vi "ClientSDO_readU32.vi"(8 "error in (no error)":errorcluster, 9 "sub_index":u8, 10 "object_index":u16, 11 "ClientSDO Ref in":refnum<k24>) -> (0 "error IO":errorcluster, 1 "ErrorCode":u32, 2 "Val":u32, 3 "ClientSDO Ref out":refnum<k24>, 4 "status":i32(ring) items=["CANOPEN_OK"=0, "CANOPEN_ERROR"=-255, "CANOPEN_ERROR_ASYNC_TRANSFER_ENABLED"=-114, "CANOPEN_ASYNC_TRANSFER"=-113, "CANOPEN_ERROR_NOT_EDS_DCF_CONFIGURED"=-112, "CANOPEN_ERROR_FILE_NOT_FOUND"=-111, "CANOPEN_ERROR_NOT_IMPLEMENTED"=-110, "CANOPEN_ERROR_NO_MESSAGE"=-109, "CANOPEN_UNSUPPORTED_BITRATE"=-108, "CANOPEN_OUT_OF_CAN_INTERFACES"=-107, "CANOPEN_ERROR_DRIVER"=-106, "CANOPEN_ERROR_HW_UNDEFINED"=-105, "CANOPEN_ERROR_HW_NOT_CONNECTED"=-104, "CANOPEN_ERROR_HW_CONNECTED"=-103, "CANOPEN_ERROR_CAN_LAYER_OVRFLOW"=-102, "CANOPEN_ERROR_CAN_LAYER"=-101, "CANOPEN_CAN_LAYER_FAILED"=-100, "CANOPEN_NODE_ID_OUT_OF_RANGE"=-15, "CANOPEN_INTERNAL_STATE_ERROR"=-14, "CANOPEN_CMD_SPEC_UNKNOWN_OR_INVALLD"=-13, "CANOPEN_ERR_DEFINED_BY_APPL"=-12, "CANOPEN_OUT_OF_MEM"=-11, "CANOPEN_REMOTE_NODE_ABORT"=-10, "CANOPEN_APP_BUF_OUT_OF_RANGE"=-9, "CANOPEN_OBJECT_MISSMATCH"=-8, "CANOPEN_BUFFER_TOO_SMALL"=-7, "CANOPEN_TOGGLE"=-6, "CANOPEN_MSG_NOT_PROCESSED"=-5, "CANOPEN_TIMEOUT"=-4, "CANOPEN_UNEXPECTED_CCS"=-3, "CANOPEN_UNEXPECTED_SCS"=-2, "CANOPEN_ARG_ERROR"=-1])   [LabVIEW 2015, in "CANOpen.lvlib"]
doc: "read DWORD from <b>client </b> using SDO protocol"
uses:
  CANOpen.lvlib
  \\Mac\Home/Desktop/imt_test_app 28-06-2012/canopenlib_cli.dll
  canopenlib_cli.dll
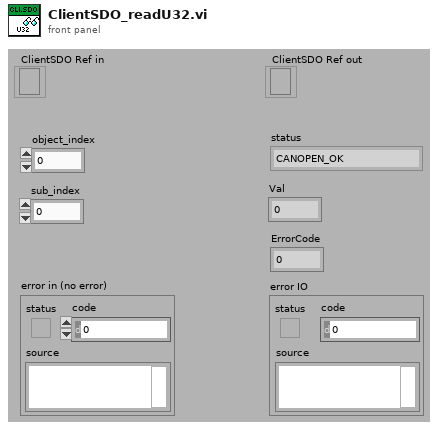
[diagram p1: front panel]
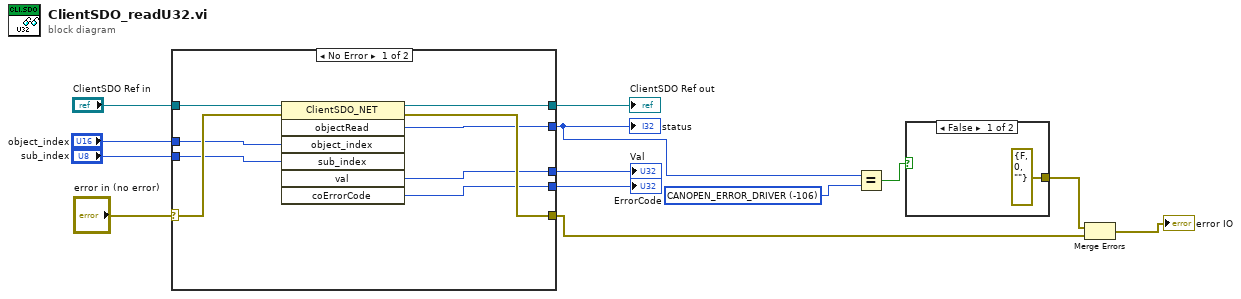
[diagram p0: block diagram]
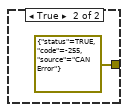
[diagram p2: hidden frame]
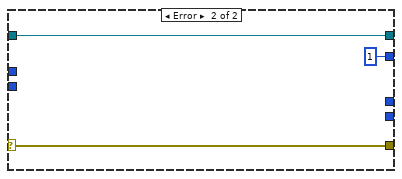
[diagram p3: hidden frame]
diagram:
  w3 = -106 items=["CANOPEN_OK"=0, "CANOPEN_ERROR"=-255, "CANOPEN_ERROR_ASYNC_TRANSFER_ENABLED"=-114, "CANOPEN_ASYNC_TRANSFER"=-113, "CANOPEN_ERROR_NOT_EDS_DCF_CONFIGURED"=-112, "CANOPEN_ERROR_FILE_NOT_FOUND"=-111, "CANOPEN_ERROR_NOT_IMPLEMENTED"=-110, "CANOPEN_ERROR_NO_MESSAGE"=-109, "CANOPEN_UNSUPPORTED_BITRATE"=-108, "CANOPEN_OUT_OF_CAN_INTERFACES"=-107, "CANOPEN_ERROR_DRIVER"=-106, "CANOPEN_ERROR_HW_UNDEFINED"=-105, "CANOPEN_ERROR_HW_NOT_CONNECTED"=-104, "CANOPEN_ERROR_HW_CONNECTED"=-103, "CANOPEN_ERROR_CAN_LAYER_OVRFLOW"=-102, "CANOPEN_ERROR_CAN_LAYER"=-101, "CANOPEN_CAN_LAYER_FAILED"=-100, "CANOPEN_NODE_ID_OUT_OF_RANGE"=-15, "CANOPEN_INTERNAL_STATE_ERROR"=-14, "CANOPEN_CMD_SPEC_UNKNOWN_OR_INVALLD"=-13, "CANOPEN_ERR_DEFINED_BY_APPL"=-12, "CANOPEN_OUT_OF_MEM"=-11, "CANOPEN_REMOTE_NODE_ABORT"=-10, "CANOPEN_APP_BUF_OUT_OF_RANGE"=-9, "CANOPEN_OBJECT_MISSMATCH"=-8, "CANOPEN_BUFFER_TOO_SMALL"=-7, "CANOPEN_TOGGLE"=-6, "CANOPEN_MSG_NOT_PROCESSED"=-5, "CANOPEN_TIMEOUT"=-4, "CANOPEN_UNEXPECTED_CCS"=-3, "CANOPEN_UNEXPECTED_SCS"=-2, "CANOPEN_ARG_ERROR"=-1] ("status 2")
  n1 = case shown="No Error" "error in (no error)" {
    selector: "error in (no error)" -> [w21 w24]
    tunnel: "ClientSDO Ref in" -> [w22 w25]
    tunnel: "object_index" -> [w20 _]
    tunnel: "sub_index" -> [w19 _]
    tunnel: [w18 w25] -> w9
    tunnel: [w17 w24] -> w4
    tunnel: [w16 1 ("objectRead")] -> w1
    tunnel: [w15 _] -> w8
    tunnel: [w14 _] -> w7
    frame No Error {
      n2 = invoke class="ClientSDO_NET" method="objectRead"(reference=w22, error in=w21, "object_index"=w20, "sub_index"=w19) -> (reference out=w18:refnum<k24>, error out=w17:errorcluster, "objectRead"=w16:i32, "val"=w15:u32, "coErrorCode"=w14:u32)  [unwired: 3 in, 2 out]
    }
    frame Error {
    }
  }
  "ClientSDO Ref out" <- w9
  "status" <- w1
  "Val" <- w8
  "ErrorCode" <- w7
  n3 = Equal?(x=w1, y=w3) -> (x = y?=w2:bool)
  n4 = case shown="False" w2 {
    tunnel: [errorcluster {"status"=FALSE, "code"=0, "source"=""} ("error constant") errorcluster {"status"=TRUE, "code"=-255, "source"="CAN Error"} ("error constant")] -> w6
    frame False {
    }
    frame True {
    }
  }
  n5 = Merge Errors(w6, w4) -> (→"error IO":errorcluster)
